vi "MainStageControl.vi"() -> ()   [LabVIEW 2019]
doc: "main user control for two dc servo and one channel 1 inertial motor"
uses:
  D:/Victor Sun/optical trap control/Kinesis/Thorlabs.MotionControl.Controls.dll
  Kinesis/Thorlabs.MotionControl.Controls.dll
  D:/Victor Sun/optical trap control/Kinesis/Thorlabs.MotionControl.KCube.InertialMotorCLI.dll
  Kinesis/Thorlabs.MotionControl.KCube.InertialMotorCLI.dll
  D:/Victor Sun/optical trap control/Kinesis/ThorLabs.MotionControl.KCube.DCServoCLI.dll
  Kinesis/ThorLabs.MotionControl.KCube.DCServoCLI.dll
panel:
  out "Position 3":i32
  in  "decrease/reverse":bool
  in  "JogStepRev in":i32=250
  in  "JogStepFwd in":i32=500
  in  "position 3":i32
  in  "Go to 3":bool
  in  "increase/forward":bool
  out "JogStepRev out":i32
  out "JogStepFwd out":i32
  in  "KCubeInertialMotorControl 3":refnum<k24>(container)
  in  "SerialNumber 3":string="97000019"
  out "Position 2":dbl format="%_6g"
  out "get absolute 2":dbl
  in  "absolute 2":dbl
  in  "Go to 2?":bool
  out "backward step size 2":dbl
  out "forward step size 2":dbl
  in  "Forward Button 2":bool
  in  "Backward Button 2":bool
  in  "relative 2":dbl=0.1
  in  "SerialNumber 2":string="27251775"
  in  "KCubeDCServoControl 2":refnum<k24>(container)
  in  "Folder path save":path
  in  "filename save":string="D:\\Victor Sun\\optical trap control\\output_test\\testposition"
  in  "start/stop write":bool
  in  "init file":bool
  out "current state":string
  out "get absolute 1":dbl
  out "backward step size":dbl
  out "forward step size":dbl
  in  "stop motors":bool
  in  "Go to 1?":bool
  in  "Backward Button":bool
  in  "Forward Button":bool
  in  "absolute 1":dbl
  in  "relative 1":dbl=0.1
  out "Position 1":dbl format="%_6g"
  in  "Stop Control Loop":bool
  in  "SerialNumber 1":string="27251750"
  in  "KCubeDCServoControl 1":refnum<k24>(container)
  # "Absolute Position Control"
  # "Relative Position Control"
  # "Data Acquisition Settings"
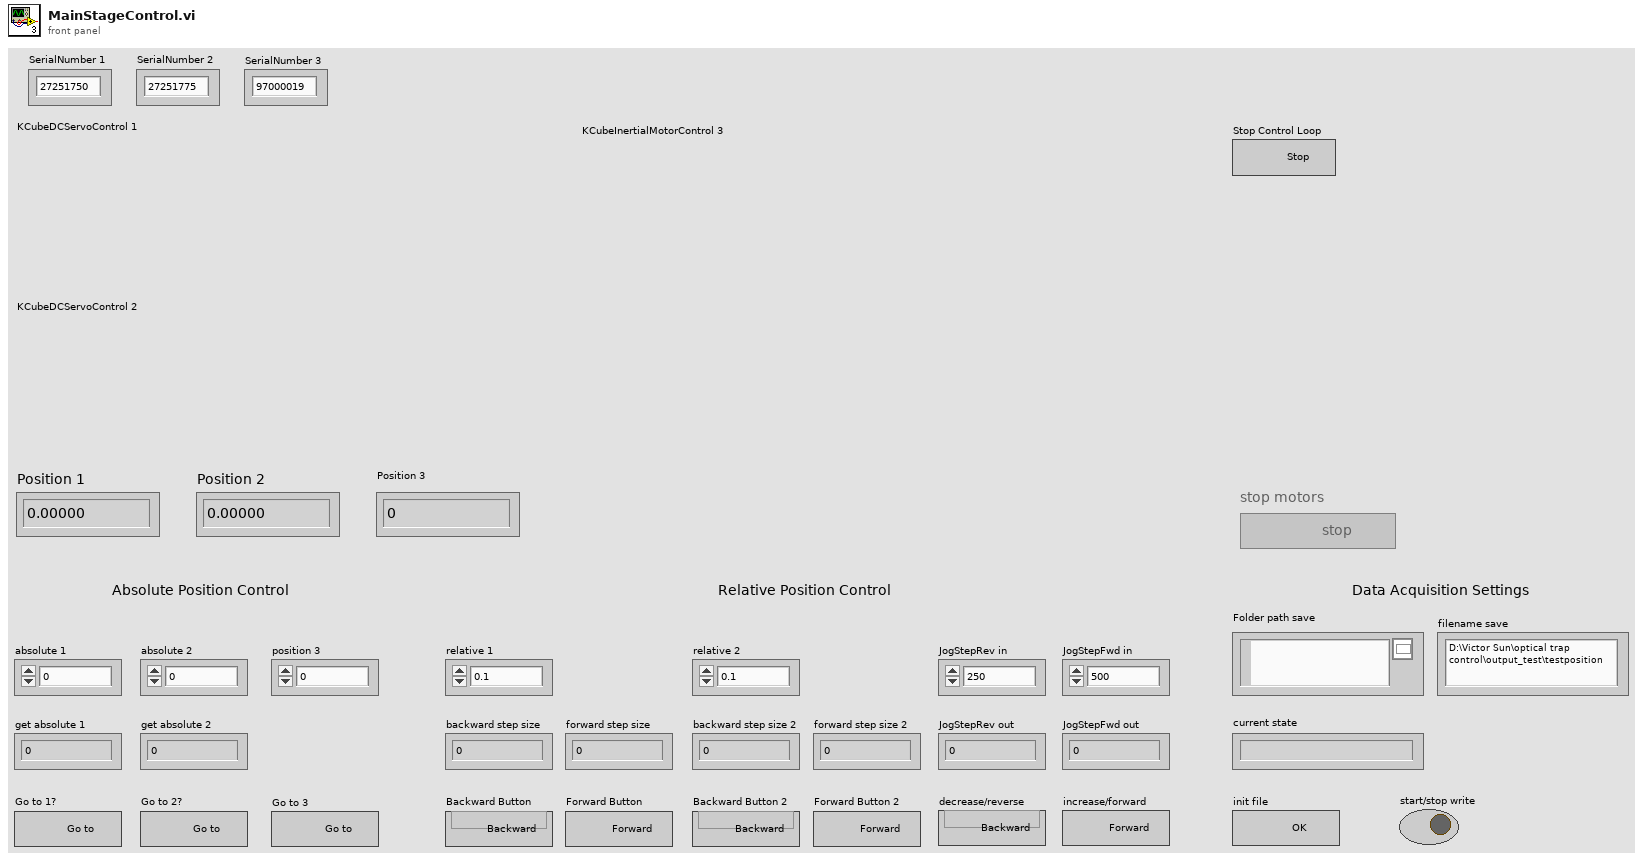
[diagram p1: front panel]
types:
  T1 = enum16{"waiting for init", "init", "waiting for write", "write", "stop"}
  T2 = enum16{"waiting for init", "init", "waiting for write", "write", "stop", ""}
  T3 = cluster{".NET Refnum out":refnum<k24>, ".NET Refnum out":refnum<k24>, ".NET Refnum out":refnum<k24>}
  T4 = cluster{"Device":refnum<k24>, "Device":refnum<k24>, "Device":refnum<k24>}
  T5 = enum8{"Enabled", "Disabled", "Disabled and Grayed Out"}
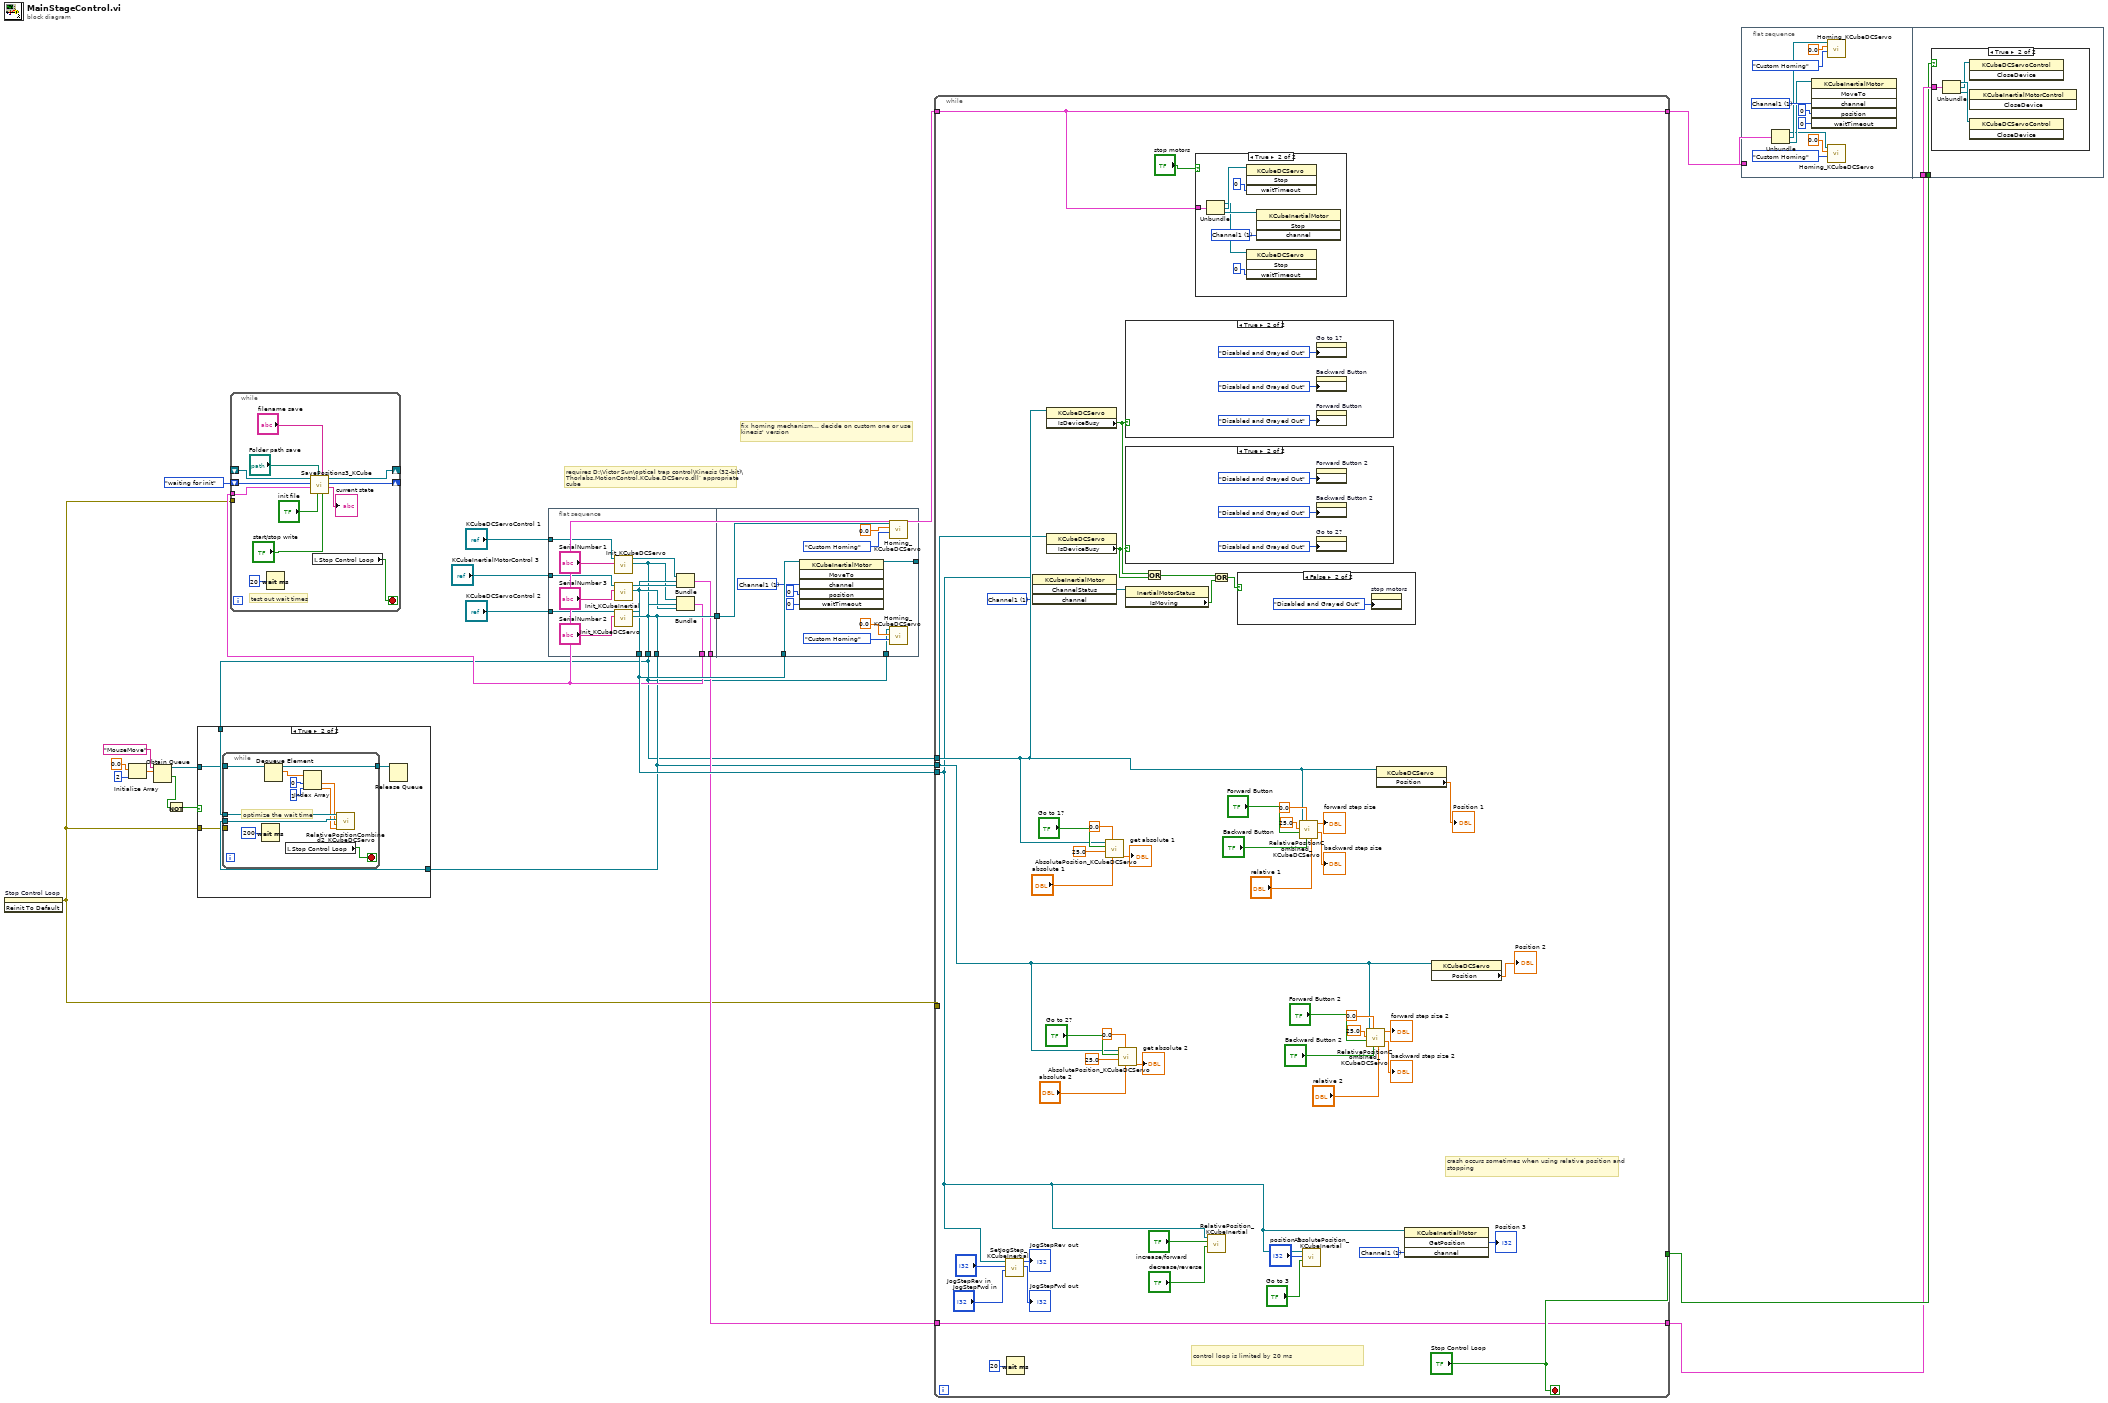
[diagram p0: block diagram]
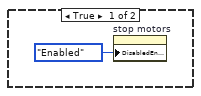
[diagram p4: hidden frame]
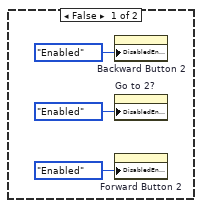
[diagram p5: hidden frame]
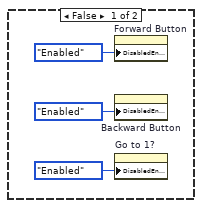
[diagram p6: hidden frame]
diagram:
  # "fix homing mechanism... decide on custom one or use kinesis' version"
  # "requires D:\\Victor Sun\\optical trap control\\Kinesis (32-bit)\\Thorlabs.MotionControl.KCube.DCServo.dll’ appropriate cube"
  n1 = invoke on="Stop Control Loop" class="Bool (strict)" method="Reinit To Default"() -> (error out=w8:errorcluster)  [unwired: 3 in, 2 out]
  n2 = Initialize Array(0.0 ("element"), 2 ("dimension size")) -> (w4:dbl[])
  n3 = Obtain Queue(name (unnamed)="MouseMove", element data type=w4) -> (queue out=w3:refnum<queue>, created new?=w1:bool)  [unwired: 3 in, 1 out]
  n4 = Not(x=w1) -> (.not. x?=w2:bool)
  n5 = case shown="True" w2 {
    tunnel: w10 -> [_ w26]
    tunnel: w9 -> [_ w25]
    tunnel: w8 -> [_ w24]
    tunnel: w3 -> [_ w23]
    frame False {
    }
    frame True {
      n6 = while {
        tunnel: w23 -> [w36]
        tunnel: w26 -> [w32]
        tunnel: w25 -> [w31]
        tunnel: [w30] -> w22
        tunnel: w24 -> [_]
        stop <- w27 stop-if-true
        # "optimize the wait time"
        n7 = Wait (ms)(milliseconds to wait=u32 200) -> ()  [unwired: 1 out]
        n8 = Dequeue Element(queue=w36) -> (queue out=w30:refnum<queue>, element=w35:dbl[])  [unwired: 2 in, 2 out]
        n9 = local read "Stop Control Loop"() -> (w27:bool)
        n10 = Index Array(array=w35, index #1=0 ("index"), index #2=1 ("index")) -> (element #1=w29:dbl, element #2=w28:dbl)
        n11 = call "RelativePositionCombined2_KCubeDCServo.vi"("element 2"=w28, "element 1"=w29, "device 2"=w32, "device 1"=w31) -> ()  [unwired: 8 in]
      }
      n12 = Release Queue(queue=w22) -> ()  [unwired: 2 in, 3 out]
    }
  }
  n13 = while {
    shift-right: [w45] -> _
    shift-left: T1."waiting for init" -> [w42]
    shift-right: [w48] -> _
    shift-left: _ -> [w47]
    tunnel: w11 -> [w39]
    tunnel: w8 -> [_]
    stop <- w38 stop-if-true
    # "test out wait times"
    n14 = Wait (ms)(milliseconds to wait=u32 20) -> ()  [unwired: 1 out]
    n15 = call "SavePositions3_KCube.vi"("start/stop write"="start/stop write", "filename save"="filename save", "init file"="init file", "Folder path save"="Folder path save", "Cluster"=w39, "Enum in"=w42, "Byte Stream File in"=w47) -> ("current state"=→"current state":string, "Enum out"=w45:T2, "Byte Stream File out"=w48:refnum<file>)  [unwired: 2 in]
    n16 = local read "Stop Control Loop"() -> (w38:bool)
  }
  n17 = flat-sequence {
    tunnel: "KCubeDCServoControl 2" -> [w63]
    tunnel: [w61] -> w19
    tunnel: [w61] -> w10
    tunnel: "KCubeDCServoControl 1" -> [w60]
    tunnel: [w50] -> w9
    tunnel: "KCubeInertialMotorControl 3" -> [w58]
    tunnel: [w57] -> w14
    tunnel: [w55] -> w11
    tunnel: [w54] -> w12
    tunnel: w19 -> [w73]
    tunnel: w9 -> [w69]
    tunnel: w14 -> [w68]
    tunnel: [w64] -> _
    frame #0 {
      n18 = call "Init_KCubeDCServo.vi"("SerialNumber"="SerialNumber 1", ".NET Refnum in"=w60) -> ("Device"=w50:refnum<k24>, ".NET Refnum out"=w51:refnum<k24>)  [unwired: 7 in, 1 out]
      n19 = call "Init_KCubeInertial.vi"("SerialNumber in"="SerialNumber 3", ".NET Refnum in"=w58) -> ("Device"=w57:refnum<k24>, ".NET Refnum out"=w53:refnum<k24>)  [unwired: 7 in, 1 out]
      n20 = call "Init_KCubeDCServo.vi"("SerialNumber"="SerialNumber 2", ".NET Refnum in"=w63) -> ("Device"=w61:refnum<k24>, ".NET Refnum out"=w52:refnum<k24>)  [unwired: 7 in, 1 out]
      n21 = Bundle(".NET Refnum out"=w51, ".NET Refnum out"=w52, ".NET Refnum out"=w53) -> (w54:T3)  [unwired: 1 in]
      n22 = Bundle("Device"=w50, "Device"=w61, "Device"=w57) -> (w55:T4)  [unwired: 1 in]
    }
    frame #1 {
      w67 = 1 items=["Channel1"=1, "Channel2"=2, "Channel3"=3, "Channel4"=4] ("channel")
      n23 = invoke class="KCubeInertialMotor" method="MoveTo"(reference=w68, "channel"=w67, "position"=0, "waitTimeout"=0) -> (reference out=w64:refnum<k24>)  [unwired: 2 in, 5 out]
      n24 = call "Homing_KCubeDCServo.vi"("Homing type"=enum16{"Custom Homing", "Kinesis Homing"}."Custom Homing", "set absolute position"=0.0 ("position"), ".NET Refnum in"=w73) -> ()  [unwired: 7 in, 2 out]
      n25 = call "Homing_KCubeDCServo.vi"("Homing type"=enum16{"Custom Homing", "Kinesis Homing"}."Custom Homing", "set absolute position"=0.0 ("position"), ".NET Refnum in"=w69) -> ()  [unwired: 7 in, 2 out]
    }
  }
  n26 = while {
    tunnel: w9 -> [w102]
    tunnel: ["Stop Control Loop"] -> w20
    tunnel: w10 -> [w95]
    tunnel: w14 -> [w77]
    tunnel: w12 -> [w76]
    tunnel: [w76] -> w17
    tunnel: w11 -> [w75]
    tunnel: [w75] -> w13
    tunnel: w8 -> [_]
    stop <- "Stop Control Loop" stop-if-true
    w80 = 1 items=["Channel1"=1, "Channel2"=2, "Channel3"=3, "Channel4"=4] ("channel")
    w84 = 1 items=["Channel1"=1, "Channel2"=2, "Channel3"=3, "Channel4"=4] ("channel")
    # "control loop is limited by 20 ms"
    # "crash occurs sometimes when using relative position and stopping"
    n27 = call "SetJogStep_KCubeInertial.vi"("JogStepFwd in"="JogStepFwd in", "JogStepRev in"="JogStepRev in", ".NET Refnum in"=w77) -> ("JogStepFwd out"=→"JogStepFwd out":i32, "JogStepRev out"=→"JogStepRev out":i32)  [unwired: 7 in]
    n28 = Wait (ms)(milliseconds to wait=u32 20) -> ()  [unwired: 1 out]
    n29 = invoke class="KCubeInertialMotor" method="ChannelStatus"(reference=w77, "channel"=w80) -> ("ChannelStatus"=w79:refnum<k24>)  [unwired: 2 in, 3 out]
    n30 = property class="KCubeDCServo"(reference=w102) -> ("IsDeviceBusy"=w94:bool)  [unwired: 1 in, 2 out]
    n31 = property class="KCubeDCServo"(reference=w95) -> ("IsDeviceBusy"=w93:bool)  [unwired: 1 in, 2 out]
    n32 = call "AbsolutePosition_KCubeDCServo.vi"("set absolute position"="absolute 1", "lower limit"=0.0, "upper limit"=25.0, "go to button"="Go to 1?", ".NET Refnum in"=w102) -> ("get absolute position"=→"get absolute 1":dbl)  [unwired: 5 in, 1 out]
    n33 = call "AbsolutePosition_KCubeDCServo.vi"("set absolute position"="absolute 2", "lower limit"=0.0, "upper limit"=25.0, "go to button"="Go to 2?", ".NET Refnum in"=w95) -> ("get absolute position"=→"get absolute 2":dbl)  [unwired: 5 in, 1 out]
    n34 = case shown="True" w94 {
      frame False {
        n35 = property on="Forward Button" class="Bool"("DisabledEnum"=T5."Enabled" ("Disabled")) -> ()  [unwired: 2 in, 2 out]
        n36 = property on="Backward Button" class="Bool"("DisabledEnum"=T5."Enabled" ("Disabled")) -> ()  [unwired: 2 in, 2 out]
        n37 = property on="Go to 1?" class="Bool"("DisabledEnum"=T5."Enabled" ("Disabled")) -> ()  [unwired: 2 in, 2 out]
      }
      frame True {
        n38 = property on="Go to 1?" class="Bool"("DisabledEnum"=T5."Disabled and Grayed Out" ("Disabled")) -> ()  [unwired: 2 in, 2 out]
        n39 = property on="Backward Button" class="Bool"("DisabledEnum"=T5."Disabled and Grayed Out" ("Disabled")) -> ()  [unwired: 2 in, 2 out]
        n40 = property on="Forward Button" class="Bool"("DisabledEnum"=T5."Disabled and Grayed Out" ("Disabled")) -> ()  [unwired: 2 in, 2 out]
      }
    }
    n41 = case shown="True" w93 {
      frame False {
        n42 = property on="Backward Button 2" class="Bool"("DisabledEnum"=T5."Enabled" ("Disabled")) -> ()  [unwired: 2 in, 2 out]
        n43 = property on="Go to 2?" class="Bool"("DisabledEnum"=T5."Enabled" ("Disabled")) -> ()  [unwired: 2 in, 2 out]
        n44 = property on="Forward Button 2" class="Bool"("DisabledEnum"=T5."Enabled" ("Disabled")) -> ()  [unwired: 2 in, 2 out]
      }
      frame True {
        n45 = property on="Forward Button 2" class="Bool"("DisabledEnum"=T5."Disabled and Grayed Out" ("Disabled")) -> ()  [unwired: 2 in, 2 out]
        n46 = property on="Backward Button 2" class="Bool"("DisabledEnum"=T5."Disabled and Grayed Out" ("Disabled")) -> ()  [unwired: 2 in, 2 out]
        n47 = property on="Go to 2?" class="Bool"("DisabledEnum"=T5."Disabled and Grayed Out" ("Disabled")) -> ()  [unwired: 2 in, 2 out]
      }
    }
    n48 = property class="InertialMotorStatus"(reference=w79) -> ("IsMoving"=w78:bool)  [unwired: 1 in, 2 out]
    n49 = Or(x=w94, y=w93) -> (x .or. y?=w82:bool)
    n50 = case shown="True" "stop motors" {
      tunnel: w75 -> [_ w143]
      frame False {
      }
      frame True {
        w144 = 1 items=["Channel1"=1, "Channel2"=2, "Channel3"=3, "Channel4"=4] ("channel")
        n51 = Unbundle(w143) -> ("Device"=w140:refnum<k24>, "Device"=w142:refnum<k24>, "Device"=w141:refnum<k24>)
        n52 = invoke class="KCubeDCServo" method="Stop"(reference=w142, "waitTimeout"=0) -> ()  [unwired: 2 in, 4 out]
        n53 = invoke class="KCubeDCServo" method="Stop"(reference=w140, "waitTimeout"=0) -> ()  [unwired: 2 in, 4 out]
        n54 = invoke class="KCubeInertialMotor" method="Stop"(reference=w141, "channel"=w144) -> ()  [unwired: 2 in, 4 out]
      }
    }
    n55 = call "RelativePosition_KCubeInertial.vi"("decrease/reverse"="decrease/reverse", "increase/forward"="increase/forward", ".NET Refnum in"=w77) -> ()  [unwired: 9 in]
    n56 = Or(x=w82, y=w78) -> (x .or. y?=w81:bool)
    n57 = case shown="False" w81 {
      frame True {
        n58 = property on="stop motors" class="Bool"("DisabledEnum"=T5."Enabled" ("Disabled")) -> ()  [unwired: 2 in, 2 out]
      }
      frame False {
        n59 = property on="stop motors" class="Bool"("DisabledEnum"=T5."Disabled and Grayed Out" ("Disabled")) -> ()  [unwired: 2 in, 2 out]
      }
    }
    n60 = call "RelativePositionCombined_KCubeDCServo.vi"("stepSize"="relative 1", "Backward Button"="Backward Button", "lower limit"=0.0, "Forward Button"="Forward Button", "upper limit"=25.0, ".NET Refnum in"=w102) -> ("backward step size"=→"backward step size":dbl, "forward step size"=→"forward step size":dbl)  [unwired: 2 in, 2 out]
    n61 = call "AbsolutePosition_KCubeInertial.vi"("go to?"="Go to 3", "set absolute position"="position 3", ".NET Refnum in"=w77) -> ()  [unwired: 9 in]
    n62 = call "RelativePositionCombined_KCubeDCServo.vi"("stepSize"="relative 2", "Backward Button"="Backward Button 2", "lower limit"=0.0, "Forward Button"="Forward Button 2", "upper limit"=25.0, ".NET Refnum in"=w95) -> ("backward step size"=→"backward step size 2":dbl, "forward step size"=→"forward step size 2":dbl)  [unwired: 2 in, 2 out]
    n63 = property class="KCubeDCServo"(reference=w102) -> ("Position"=→"Position 1":dbl)  [unwired: 1 in, 2 out]
    n64 = invoke class="KCubeInertialMotor" method="GetPosition"(reference=w77, "channel"=w84) -> ("GetPosition"=→"Position 3":i32)  [unwired: 2 in, 3 out]
    n65 = property class="KCubeDCServo"(reference=w95) -> ("Position"=→"Position 2":dbl)  [unwired: 1 in, 2 out]
  }
  n66 = flat-sequence {
    tunnel: w13 -> [w150]
    tunnel: w20 -> [w158]
    tunnel: w17 -> [w159]
    frame #0 {
      w153 = 1 items=["Channel1"=1, "Channel2"=2, "Channel3"=3, "Channel4"=4] ("channel")
      n67 = Unbundle(w150) -> ("Device"=w147:refnum<k24>, "Device"=w148:refnum<k24>, "Device"=w149:refnum<k24>)
      n68 = invoke class="KCubeInertialMotor" method="MoveTo"(reference=w149, "channel"=w153, "position"=0, "waitTimeout"=0) -> ()  [unwired: 2 in, 6 out]
      n69 = call "Homing_KCubeDCServo.vi"("Homing type"=enum16{"Custom Homing", "Kinesis Homing"}."Custom Homing", "set absolute position"=0.0 ("position"), ".NET Refnum in"=w148) -> ()  [unwired: 7 in, 2 out]
      n70 = call "Homing_KCubeDCServo.vi"("Homing type"=enum16{"Custom Homing", "Kinesis Homing"}."Custom Homing", "set absolute position"=0.0 ("position"), ".NET Refnum in"=w147) -> ()  [unwired: 7 in, 2 out]
    }
    frame #1 {
      n71 = case shown="True" w158 {
        tunnel: w159 -> [_ w163]
        frame False {
        }
        frame True {
          n72 = Unbundle(w163) -> (".NET Refnum out"=w162:refnum<k24>, ".NET Refnum out"=w161:refnum<k24>, ".NET Refnum out"=w160:refnum<k24>)
          n73 = invoke class="KCubeDCServoControl" method="CloseDevice"(reference=w161) -> ()  [unwired: 2 in, 3 out]
          n74 = invoke class="KCubeInertialMotorControl" method="CloseDevice"(reference=w160) -> ()  [unwired: 2 in, 3 out]
          n75 = invoke class="KCubeDCServoControl" method="CloseDevice"(reference=w162) -> ()  [unwired: 2 in, 3 out]
        }
      }
    }
  }
